vi "sweep-values-sub.vi"(4 "Forward/Reverse":bool, 5 "Point Number":i32, 6 "Step Size":dbl format="%.2f", 7 "Sweep Stop":dbl format="%.2f", 8 "Sweep Start":dbl format="%.2f") -> (1 "Active":bool, 3 "Output":dbl format="%.2f")   [LabVIEW 2018]
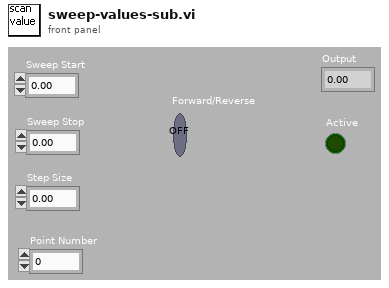
[diagram p1: front panel]
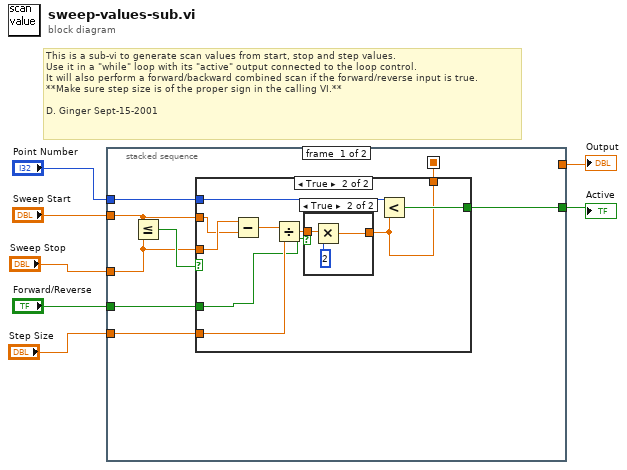
[diagram p0: block diagram]
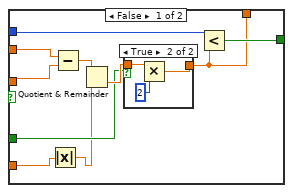
[diagram p2: hidden frame]
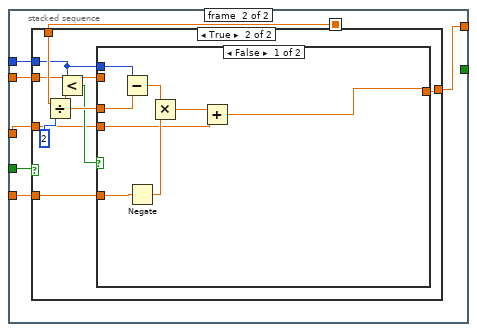
[diagram p5: hidden frame]
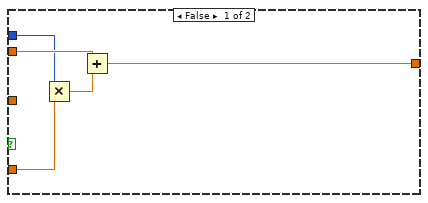
[diagram p6: hidden frame]
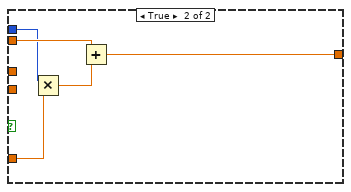
[diagram p7: hidden frame]
diagram:
  # "This is a sub-vi to generate scan values from start, stop and step values.\nUse it in a \"while\" loop with its \"active\" output connected to the loop control.\nIt will also perform a forward/backward combined scan if the forward/reverse input is true.\n**Make sure step size is of the proper sign in the calling VI.**\n\nD. Ginger Sept-15-2001"
  n1 = stacked-sequence {
    seq-local: [w8 _] -> [_ w44]
    tunnel: "Sweep Start" -> [w13 w48]
    tunnel: "Sweep Stop" -> [w14 w43]
    tunnel: "Step Size" -> [w12 w47]
    tunnel: "Point Number" -> [w11 w46]
    tunnel: "Forward/Reverse" -> [w10 w49]
    tunnel: [w9 _] -> w2
    tunnel: [_ w45] -> w1
    frame #0 {
      n2 = Less Or Equal?(x=w13, y=w14) -> (x <= y?=w15:bool)
      n3 = case shown="True" w15 {
        tunnel: w14 -> [w20 w38]
        tunnel: w13 -> [w19 w37]
        tunnel: w12 -> [w17 w35]
        tunnel: w11 -> [w22 w34]
        tunnel: w10 -> [w21 w32]
        tunnel: [w25 w31] -> w9
        tunnel: [w18 w30] -> w8
        frame False {
          n4 = Absolute Value(x=w17) -> (abs(x)=w16:dbl)
          n5 = Subtract(x=w19, y=w20) -> (x-y=w23:dbl)
          n6 = Quotient & Remainder(x=w23, y=w16) -> (floor(x/y)=w24:dbl)  [unwired: 1 out]
          n7 = case shown="True" w21 {
            tunnel: [w26 w29] -> w18
            tunnel: w24 -> [w26 w28]
            frame False {
            }
            frame True {
              n8 = Multiply(x=w28, y=2) -> (x*y=w29:dbl)
            }
          }
          n9 = Less?(x=w22, y=w18) -> (x < y?=w25:bool)
        }
        frame True {
          n10 = Subtract(x=w38, y=w37) -> (x-y=w36:dbl)
          n11 = Divide(x=w36, y=w35) -> (x/y=w33:dbl)
          n12 = case shown="True" w32 {
            tunnel: [w39 w42] -> w30
            tunnel: w33 -> [w39 w41]
            frame False {
            }
            frame True {
              n13 = Multiply(x=w41, y=2) -> (x*y=w42:dbl)
            }
          }
          n14 = Less?(x=w34, y=w30) -> (x < y?=w31:bool)
        }
      }
    }
    frame #1 {
      n15 = case shown="True" w49 {
        tunnel: w48 -> [w54 w59]
        tunnel: w47 -> [w53 w58]
        tunnel: w46 -> [w51 w57]
        tunnel: [w50 w56] -> w45
        tunnel: w44 -> [_ w62]
        tunnel: w43 -> [_ w55]
        frame False {
          n16 = Multiply(x=w51, y=w53) -> (x*y=w52:dbl)
          n17 = Add(x=w54, y=w52) -> (x+y=w50:dbl)
        }
        frame True {
          n18 = Divide(x=w62, y=2) -> (x/y=w61:dbl)
          n19 = Less?(x=w57, y=w61) -> (x < y?=w60:bool)
          n20 = case shown="False" w60 {
            tunnel: w59 -> [_ w76]
            tunnel: w58 -> [w68 w75]
            tunnel: w57 -> [w71 w74]
            tunnel: [w64 w72] -> w56
            tunnel: w61 -> [w70 _]
            tunnel: w55 -> [w65 _]
            frame False {
              n21 = Subtract(x=w71, y=w70) -> (x-y=w69:dbl)
              n22 = Negate(x=w68) -> (-x=w67:dbl)
              n23 = Multiply(x=w69, y=w67) -> (x*y=w66:dbl)
              n24 = Add(x=w66, y=w65) -> (x+y=w64:dbl)
            }
            frame True {
              n25 = Multiply(x=w74, y=w75) -> (x*y=w73:dbl)
              n26 = Add(x=w76, y=w73) -> (x+y=w72:dbl)
            }
          }
        }
      }
    }
  }
  "Output" <- w1
  "Active" <- w2
